vi "reset-class-data.vi"(8 "error in (no error)":errorcluster, 11 "CANtable in":refnum<class "bFrameIO.lvclass">) -> (0 "error out":errorcluster, 3 "CANtable out":refnum<class "bFrameIO.lvclass">)   [LabVIEW 2015, in "bFrameIO.lvclass"]
uses:
  bFrameIO.lvclass
  controls/input-states.ctl
  bFrameIO.lvclass/bFrameIO.ctl
  wrt-fi-state.vi
  class.can.table/bAPPdata.lvclass
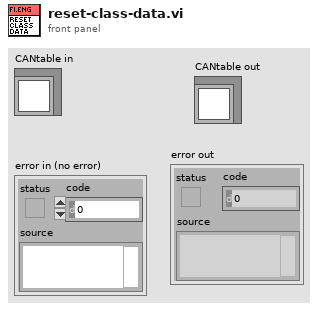
[diagram p1: front panel]
types:
  T1 = typedef "bFrameIO.lvclass/input-states.ctl" = enum16{"idle", "start", "run", "stop", "exit"}
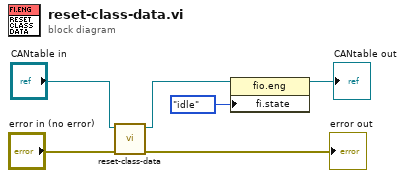
[diagram p0: block diagram]
diagram:
  n1 = call-parent "reset-class-data.vi"("error in (no error)"="error in (no error)", "CANtable in"="CANtable in") -> ("error out"=→"error out":errorcluster, "CANtable out"=w5:refnum<class "bFrameIO.lvclass">)  [unwired: 8 in]
  n2 = property class="fio.eng"(reference=w5, "fi.state"=input-states."idle") -> (reference out=→"CANtable out":refnum<class "bFrameIO.lvclass">)  [unwired: 1 in, 1 out]
